vi "VF_IQenvelope.vi"() -> ()   [LabVIEW 2018]
uses:
  <vilib>/Analysis/3filter.llb/Filter Passband Type.ctl
  <vilib>/Analysis/2dsp.llb/1D Convolution (DBL).vi
  <vilib>/measure/maspectr.llb/FFT Power Spectrum and PSD for 1 Chan.vi
  <vilib>/measure/maspectr.llb/FFT Power Spectrum and PSD for 1 Chan (CDB).vi
  <vilib>/Analysis/3filter.llb/Butterworth Filter (DBL).vi
  <vilib>/rtlsdr/rtlsdr.lvlib
  <vilib>/measure/NI_MAPro.lvlib
  <vilib>/Analysis/NI_AALBase.lvlib
  <vilib>/Analysis/NI_AALPro.lvlib
panel:
  in  "exponencial":dbl
  in  "modulo":dbl
  in  "order":i32=2
  in  "low cutoff freq: fl":dbl=0.12500000000000006 format="%0.4f"
  out "f0":dbl
  out "x+y":i32
  out "Power Spectrum 2":cluster{"f0":dbl, "df":dbl, "magnitude":dbl[]}(graph)
  out "Power Spectrum":cluster{"f0":dbl, "df":dbl, "magnitude":dbl[]}[](graph)
  out "Center Frequency":dbl
  in  "config":bool
  in  "Number Of Samples":i32
  in  "Center Frequency":u32
  in  "Sample Rate":u32
  out "function return":i32
  in  "Device Index":u32
  out "Device USB Strings":T1
  out "DeviceRefnum Out":u64
  in  "stop":bool
  out "Device Count":u32
  # "1"
  # "2228"
  # "50"
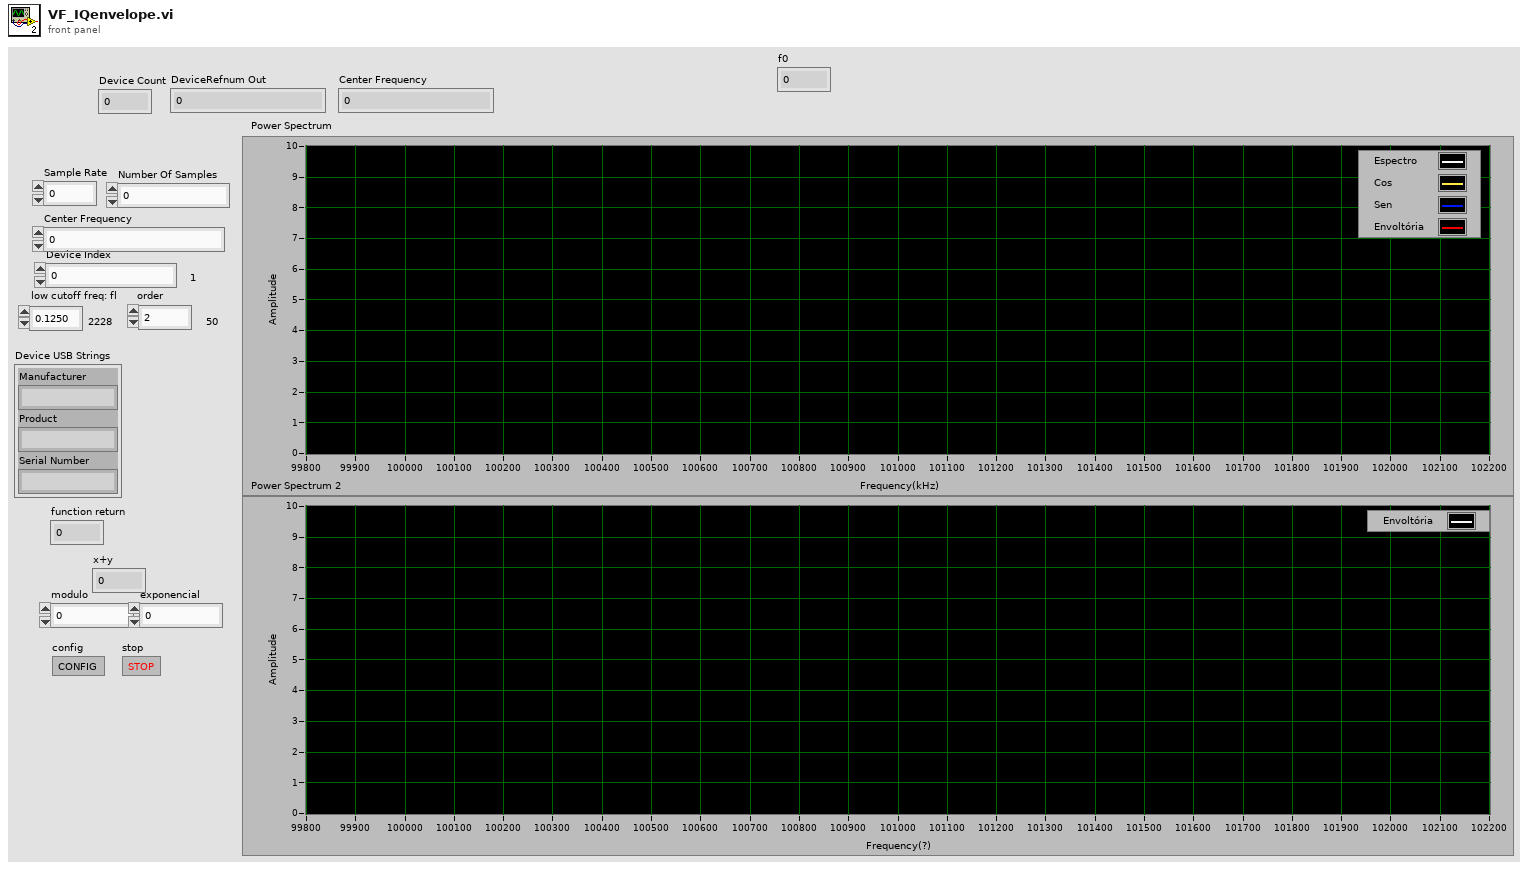
[diagram p1: front panel]
types:
  T1 = cluster{"Manufacturer":string, "Product":string, "Serial Number":string}
  T2 = typedef "NI_AALBase.lvlib/Filter Passband Type.ctl" = enum32{"Lowpass", "Highpass", "Bandpass", "Bandstop"}
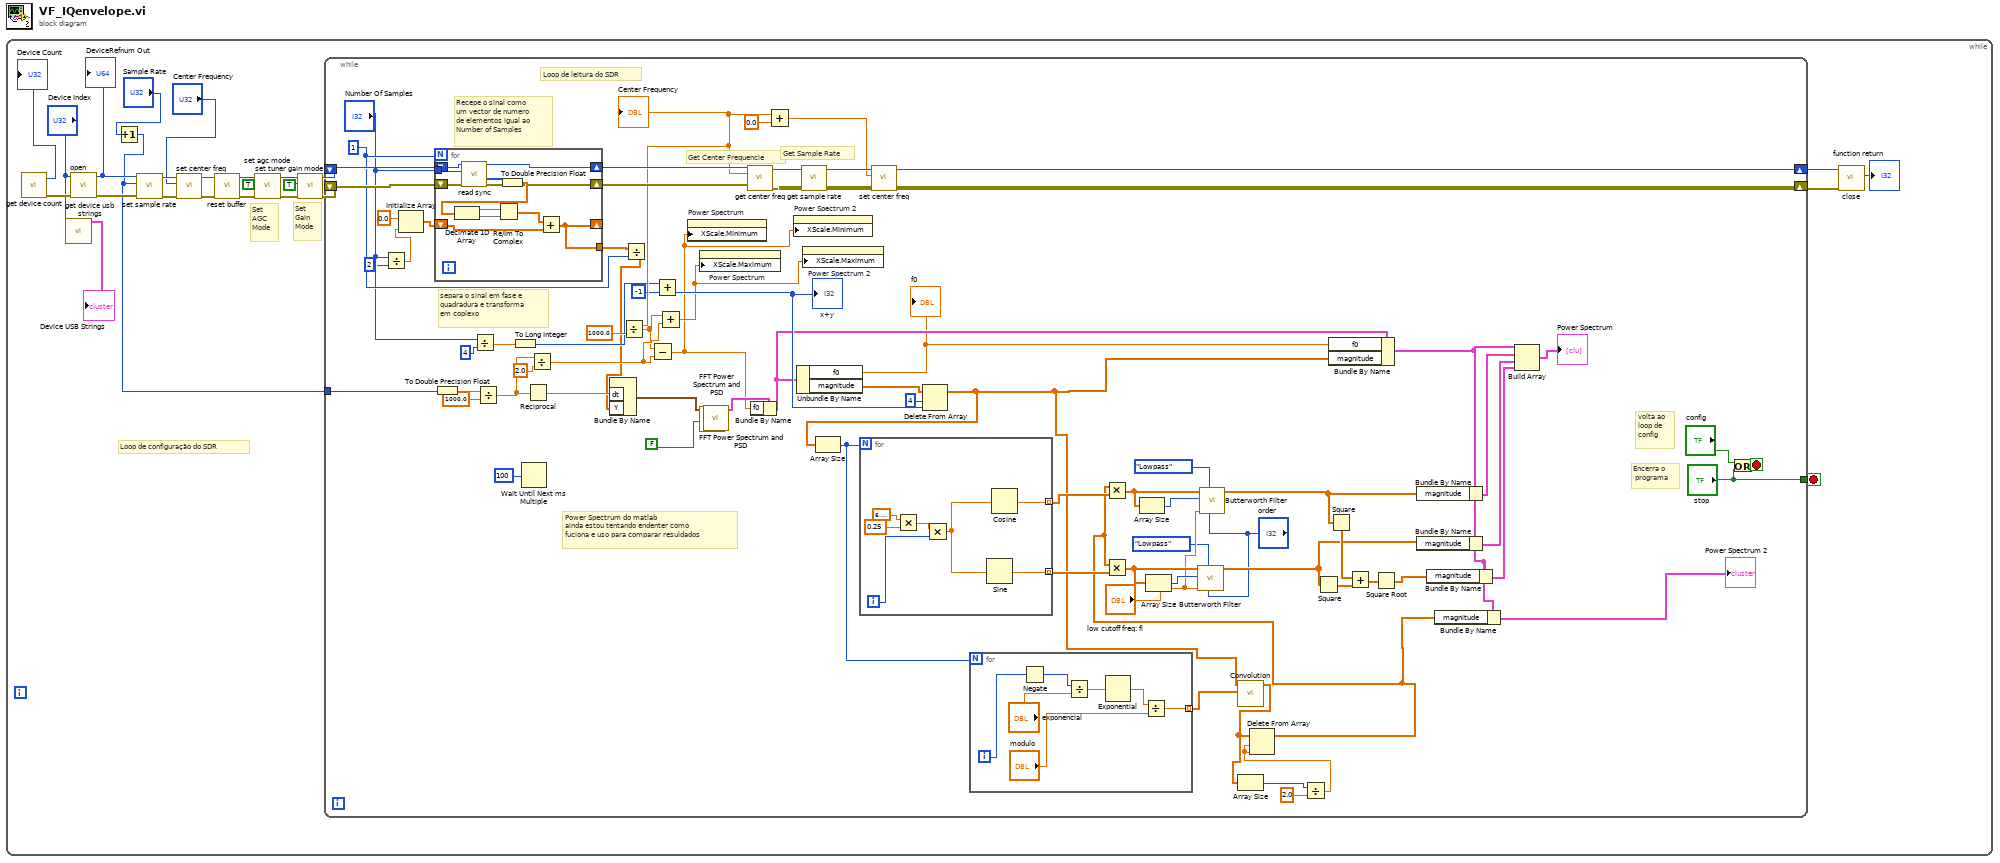
[diagram p0: block diagram]
diagram:
  n1 = while {
    stop <- w5 stop-if-true
    # "Set\nGain\nMode"
    # "Set\nAGC\nMode"
    # "Loop de configuração do SDR"
    n2 = call <vilib>:"get device count.vi"() -> ("error out"=w24:errorcluster, "Device Count"=→"Device Count":u32)  [unwired: 10 in]
    n3 = call <vilib>:"get device usb strings.vi"("Device Index"="Device Index") -> ("Device USB Strings"=→"Device USB Strings":T1)  [unwired: 8 in, 2 out]
    n4 = call <vilib>:"open.vi"("error in (no error)"=w24, "Device Index"="Device Index") -> ("error out"=w20:errorcluster, "DeviceRefnum Out"=w19:u64)  [unwired: 6 in]
    "DeviceRefnum Out" <- w19
    n5 = Increment(x="Sample Rate") -> (x+1=w1:u32)
    n6 = call <vilib>:"set sample rate.vi"("error in (no error)"=w20, "Sample Rate"=w1, "DeviceRefnum"=w19) -> ("error out"=w18:errorcluster, "DeviceRefnum Out"=w17:u64)  [unwired: 6 in, 1 out]
    n7 = call <vilib>:"set center freq.vi"("error in (no error)"=w18, "Center Frequency"="Center Frequency", "DeviceRefnum"=w17) -> ("error out"=w16:errorcluster, "DeviceRefnum Out"=w15:u64)  [unwired: 6 in, 1 out]
    n8 = call <vilib>:"reset buffer.vi"("error in (no error)"=w16, "DeviceRefnum"=w15) -> ("error out"=w14:errorcluster, "DeviceRefnum Out"=w13:u64)  [unwired: 7 in, 1 out]
    n9 = call <vilib>:"set agc mode.vi"("error in (no error)"=w14, "AGC Enable"=TRUE, "DeviceRefnum"=w13) -> ("error out"=w12:errorcluster, "DeviceRefnum Out"=w11:u64)  [unwired: 6 in, 1 out]
    n10 = call <vilib>:"set tuner gain mode.vi"("error in (no error)"=w12, "AutoGain"=TRUE ("AGC Enable"), "DeviceRefnum"=w11) -> ("error out"=w9:errorcluster, "DeviceRefnum Out"=w8:u64)  [unwired: 6 in, 1 out]
    n11 = while {
      shift-right: [w87] -> w6
      shift-left: w8 -> [w102]
      shift-right: [w86] -> w7
      shift-left: w9 -> [w103]
      tunnel: ["stop"] -> w5
      tunnel: w1 -> [w85]
      stop <- w100 stop-if-true
      w68 = 1
      # "separa o sinal em fase e\nquadradura e transforma\nem coplexo"
      # "Recepe o sinal como\num vector de numero\nde elementos igual ao\nNumber of Samples"
      # "Encerra o\n programa"
      # "volta ao\nloop de \nconfig"
      # "Power Spectrum do matlab\nainda estou tentando endenter como \nfuciona e uso para comparar resuldados"
      # "Get Center Frequencie"
      # "Get Sample Rate"
      # "Loop de leitura do SDR"
      n12 = Divide(x="Number Of Samples", y=2) -> (x/y=w63:dbl)
      n13 = Initialize Array(0.0 ("element"), w63) -> (w65:dbl[])
      n14 = for {
        N: w68 -> [_]
        tunnel: "Number Of Samples" -> [w124]
        shift-right: [w123] -> w93
        shift-left: w103 -> [w129]
        shift-right: [w125] -> w97
        shift-left: w102 -> [w128]
        shift-right: [w119] -> _
        shift-left: w65 -> [w118]
        tunnel: [w119] -> w66
        n15 = call <vilib>:"read sync.vi"("error in (no error)"=w129, "Number Of Samples"=w124, "DeviceRefnum"=w128) -> ("error out"=w123:errorcluster, "Sample Buffer"=w126:u8[], "DeviceRefnum Out"=w125:u64)  [unwired: 5 in, 1 out]
        n16 = To Double Precision Float(number=w126) -> (double precision float=w127:dbl[])
        n17 = Decimate 1D Array(w127) -> (w122:dbl[], w121:dbl[])
        n18 = Re/Im To Complex(1:w121, 2:w122) -> (0:w120:cdb[])
        n19 = Add(x=w120, y=w118) -> (x+y=w119:cdb[])
      }
      n20 = To Double Precision Float(number=w85) -> (double precision float=w77:dbl)
      n21 = Divide(x="Number Of Samples", y=4) -> (x/y=w95:dbl)
      n22 = Divide(x=w77, y=1000.0) -> (x/y=w81:dbl)
      n23 = To Long Integer(number=w95) -> (32bit integer=w72:i32)
      n24 = Wait Until Next ms Multiple(millisecond multiple=u32 100) -> ()  [unwired: 1 out]
      n25 = Reciprocal(x=w81) -> (1/x=w83:dbl)
      n26 = Divide(x=w81, y=2.0) -> (x/y=w70:dbl)
      n27 = Divide(x=w66, y=w68) -> (x/y=w67:cdb[])
      n28 = Bundle By Name("dt"=w83, "Y"=w67) -> (w84:waveform(cdb))  [unwired: 1 in]
      n29 = Add(x=w72, y=-1) -> (x+y=w73:i32)
      "x+y" <- w73
      n30 = call-poly <vilib>:"FFT Power Spectrum and PSD.vi"() -> ()  [unwired: 8 in, 4 out]
      n31 = call-poly <vilib>:"FFT Power Spectrum and PSD.vi"("dB On (F)"=FALSE, "time signal"=w84) -> ("Power Spectrum / PSD"=w76:cluster{"f0":dbl, "df":dbl, "magnitude":dbl[]})  [unwired: 6 in, 3 out]
      n32 = call <vilib>:"get center freq.vi"("error in (no error)"=w93, "DeviceRefnum"=w97) -> ("error out"=w92:errorcluster, "Center Frequency"=w79:dbl, "DeviceRefnum Out"=w94:u64)  [unwired: 7 in]
      "Center Frequency" <- w79
      n33 = Divide(x=w79, y=1000.0) -> (x/y=w69:dbl)
      n34 = Subtract(x=w69, y=w70) -> (x-y=w44:dbl)
      n35 = Add(x=w69, y=w70) -> (x+y=w45:dbl)
      n36 = property on="Power Spectrum" class="WFGraph (strict)"("XScale.Minimum"=w44) -> ()  [unwired: 2 in, 2 out]
      n37 = property on="Power Spectrum" class="WFGraph (strict)"("XScale.Maximum"=w45) -> ()  [unwired: 2 in, 2 out]
      n38 = Bundle By Name(cluster=w76, "f0"=w44) -> (w60:cluster{"f0":dbl, "df":dbl, "magnitude":dbl[]})
      n39 = Add(x=w79, y=0.0) -> (x+y=w88:dbl)
      n40 = property on="Power Spectrum 2" class="WFGraph (strict)"("XScale.Minimum"=w44) -> ()  [unwired: 2 in, 2 out]
      n41 = Unbundle By Name(w60) -> ("f0"=w59:dbl, "magnitude"=w75:dbl[])
      "f0" <- w59
      n42 = call <vilib>:"get sample rate.vi"("error in (no error)"=w92, "DeviceRefnum"=w94) -> ("error out"=w91:errorcluster, "DeviceRefnum Out"=w90:u64)  [unwired: 7 in, 1 out]
      n43 = property on="Power Spectrum 2" class="WFGraph (strict)"("XScale.Maximum"=w45) -> ()  [unwired: 2 in, 2 out]
      n44 = call <vilib>:"set center freq.vi"("error in (no error)"=w91, "Center Frequency"=w88, "DeviceRefnum"=w90) -> ("error out"=w86:errorcluster, "DeviceRefnum Out"=w87:u64)  [unwired: 6 in, 1 out]
      n45 = Delete From Array(array=w75, length=4, index=w73) -> (array with subset deleted=w27:dbl[])  [unwired: 1 out]
      n46 = Array Size(array=w27) -> (size(s)=w37:i32)
      n47 = for {
        N: w37 -> [_]
        tunnel: [w116] -> w43 mode=indexing
        tunnel: [w115] -> w42 mode=indexing
        i -> [w111]
        n48 = Multiply(x=6.283185307179586, y=0.25) -> (x*y=w114:dbl)
        n49 = Multiply(x=w114, y=w111) -> (x*y=w112:dbl)
        n50 = Sine(x=w112) -> (sin(x)=w115:dbl)
        n51 = Cosine(x=w112) -> (cos(x)=w116:dbl)
      }
      n52 = for {
        N: w37 -> [_]
        tunnel: [w104] -> w32 mode=indexing
        i -> [w110]
        n53 = Negate(x=w110) -> (-x=w109:i32)
        n54 = Divide(x=w109, y="exponencial") -> (x/y=w107:dbl)
        n55 = Exponential(1:w107) -> (0:w106:dbl)
        n56 = Divide(x=w106, y="modulo") -> (x/y=w104:dbl)
      }
      n57 = call-poly <vilib>:"Convolution.vi"("Y"=w32, "X"=w27) -> ("X * Y"=w33:dbl[])  [unwired: 8 in, 1 out]
      n58 = Array Size(array=w33) -> (size(s)=w35:i32)
      n59 = Divide(x=w35, y=2.0) -> (x/y=w34:dbl)
      n60 = Delete From Array(array=w33, length=w34, index=w34) -> (array with subset deleted=w26:dbl[])  [unwired: 1 out]
      n61 = Multiply(x=w26, y=w43) -> (x*y=w49:dbl[])
      n62 = Multiply(x=w26, y=w42) -> (x*y=w47:dbl[])
      n63 = Array Size(array=w49) -> (size(s)=w48:i32)
      n64 = Array Size(array=w47) -> (size(s)=w41:i32)
      n65 = call-poly <vilib>:"Butterworth Filter.vi"("order"="order", "filter type"=Filter_Passband_Type."Lowpass", "low cutoff freq: fl"="low cutoff freq: fl", "sampling freq: fs"=w41, "X"=w47) -> ("Filtered X"=w51:dbl[])  [unwired: 3 in, 1 out]
      n66 = call-poly <vilib>:"Butterworth Filter.vi"("order"="order", "filter type"=Filter_Passband_Type."Lowpass", "low cutoff freq: fl"="low cutoff freq: fl", "sampling freq: fs"=w48, "X"=w49) -> ("Filtered X"=w52:dbl[])  [unwired: 3 in, 1 out]
      n67 = Square(x=w51) -> (x^2=w56:dbl[])
      n68 = Square(x=w52) -> (x^2=w57:dbl[])
      n69 = Bundle By Name(cluster=w60, "f0"=w59, "magnitude"=w27) -> (w30:cluster{"f0":dbl, "df":dbl, "magnitude":dbl[]})
      n70 = Add(x=w57, y=w56) -> (x+y=w55:dbl[])
      n71 = Square Root(x=w55) -> (sqrt(x)=w28:dbl[])
      n72 = Bundle By Name(cluster=w30, "magnitude"=w52) -> (w53:cluster{"f0":dbl, "df":dbl, "magnitude":dbl[]})
      n73 = Bundle By Name(cluster=w30, "magnitude"=w51) -> (w46:cluster{"f0":dbl, "df":dbl, "magnitude":dbl[]})
      n74 = Bundle By Name(cluster=w30, "magnitude"=w28) -> (w31:cluster{"f0":dbl, "df":dbl, "magnitude":dbl[]})
      n75 = Bundle By Name(cluster=w30, "magnitude"=w26) -> (→"Power Spectrum 2":cluster{"f0":dbl, "df":dbl, "magnitude":dbl[]})
      n76 = Build Array(w30, w53, w46, w31) -> (→"Power Spectrum":cluster{"f0":dbl, "df":dbl, "magnitude":dbl[]}[])
      n77 = Or(x="config", y="stop") -> (x .or. y?=w100:bool)
    }
    n78 = call <vilib>:"close.vi"("error in (no error)"=w7, "DeviceRefnum"=w6) -> ("function return"=→"function return":i32)  [unwired: 8 in, 1 out]
  }
